vi "AbortReachGoal_get.vi"(8 "error in (no error)":errorcluster) -> (0 "error out":errorcluster, 2 "Abort":bool)   [LabVIEW 2009, in "Main.lvlib" / "MainVariables.lvlib"]
doc: "Get value of AbortReachGoal variable"
uses:
  MainVariables.lvlib
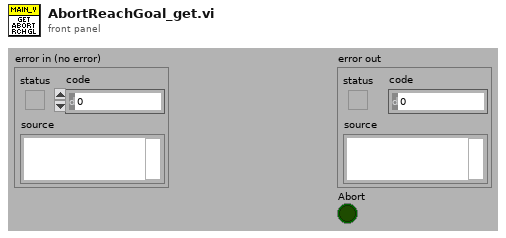
[diagram p1: front panel]
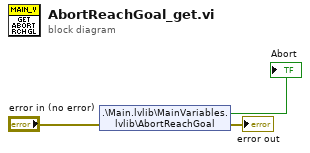
[diagram p0: block diagram]
diagram:
  n1 = shared-variable ".\\Main.lvlib\\MainVariables.lvlib\\AbortReachGoal"(error in="error in (no error)") -> (→"Abort":bool, error out=→"error out":errorcluster)
